vi "AIT 1553 - Report License Status.vi"(0 "Device Item Ref in":T1 format="%.0x", 5 "activation successful?":bool, 11 "error in (no error)":errorcluster) -> (15 "error out":errorcluster)   [LabVIEW 2013, in "AIT 1553 Custom Device.lvlib"]
doc: "Reports status of license status back to VeriStand"
uses:
  AIT 1553 Custom Device.lvlib
  <vilib>/NI Veristand/Custom Device API/Custom Device Item Ref.ctl
  <vilib>/NI Veristand/Custom Device API/Custom Device API.lvlib
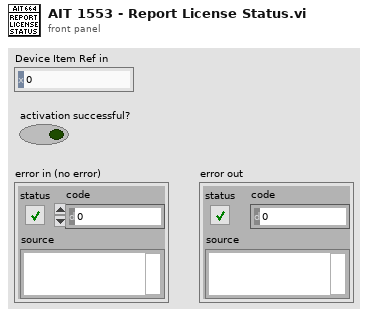
[diagram p1: front panel]
types:
  T1 = typedef "Custom Device API.lvlib/Custom Device Item Ref.ctl" = u64
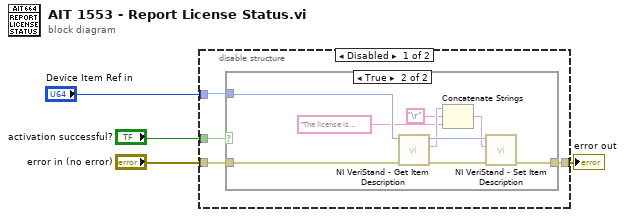
[diagram p0: block diagram]
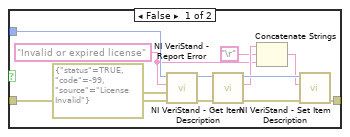
[diagram p2: hidden frame]
diagram:
  n1 = disable-structure shown="Disabled" {
    disable-tunnel: "error in (no error)" -> [w8 w30]
    disable-tunnel: [w7 w30] -> w2
    disable-tunnel: "Device Item Ref in" -> [w6 _]
    disable-tunnel: "activation successful?" -> [w5 _]
    frame Disabled {
      n2 = case shown="True" w5 {
        tunnel: w6 -> [w20 w22]
        tunnel: w8 -> [w19 w23]
        tunnel: [w13 w24] -> w7
        frame False {
          w11 = "Invalid or expired license" ("Error ID")
          n3 = call <vilib>:"NI VeriStand - Report Error.vi"("error in (no error)"=w19, "New Error"=errorcluster {"status"=TRUE, "code"=-99, "source"="License Invalid"}, "Error ID"=w11, "Node Ref in"=w20) -> ("error out"=w17:errorcluster, "Node Ref out"=w16:T1)  [unwired: 6 in]
          n4 = call <vilib>:"NI VeriStand - Get Item Description.vi"("error in (no error)"=w17, "Item Ref in"=w16) -> ("error out"=w14:errorcluster, "Description"=w12:string, "Item Ref out"=w15:T1)  [unwired: 6 in, 1 out]
          n5 = Concatenate Strings(w12, "\r", w11) -> (w9:string)
          n6 = call <vilib>:"NI VeriStand - Set Item Description.vi"("error in (no error)"=w14, "Description"=w9, "Item Ref in"=w15) -> ("error out"=w13:errorcluster)  [unwired: 6 in, 2 out]
        }
        frame True {
          n7 = call <vilib>:"NI VeriStand - Get Item Description.vi"("error in (no error)"=w23, "Item Ref in"=w22) -> ("error out"=w25:errorcluster, "Description"=w28:string, "Item Ref out"=w29:T1)  [unwired: 6 in, 1 out]
          n8 = Concatenate Strings(w28, "\r", "The license is either valid or in an evaluation mode." ("string")) -> (w26:string)
          n9 = call <vilib>:"NI VeriStand - Set Item Description.vi"("error in (no error)"=w25, "Description"=w26, "Item Ref in"=w29) -> ("error out"=w24:errorcluster)  [unwired: 6 in, 2 out]
        }
      }
    }
    frame Enabled {
      # "would display a message in the discription\nevery time device is accessed, deemed not needed\npop up should be sufficient"
    }
  }
  "error out" <- w2
